vi "Write Bytes.vi"(8 "error in (no error)":errorcluster {"code" format="%.0x"}, 9 "Buffer":u32[](array[numeric])=[0], 10 "Count":i64 format="%.0g", 11 "instrument handle":refnum<k15>) -> (0 "error out":errorcluster {"code" format="%.0x"}, 2 "ReturnCount":i64, 3 "instrument handle out":refnum<k15>)   [LabVIEW 2020, in "Keysight DAQ970.lvlib"]
doc: "Write an array of bytes to the device."
uses:
  Keysight DAQ970.lvlib
  KtDAQ970.dll
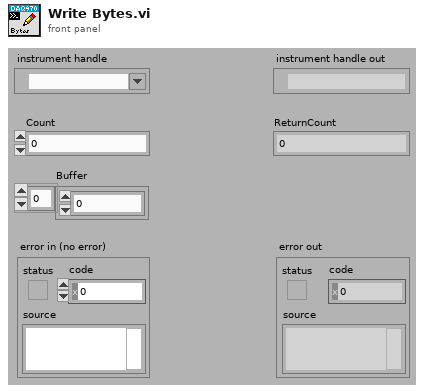
[diagram p1: front panel]
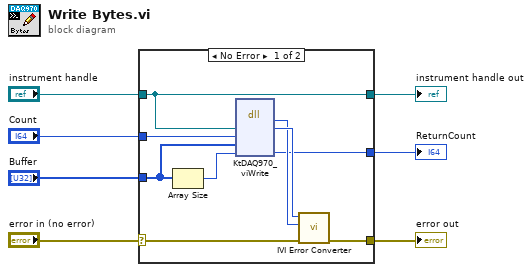
[diagram p0: block diagram]
diagram:
  n1 = case shown="No Error" "error in (no error)" {
    selector: "error in (no error)" -> [w14 w18]
    tunnel: [w13 w18] -> w7
    tunnel: "instrument handle" -> [w10 w17]
    tunnel: "Count" -> [w12 _]
    tunnel: "Buffer" -> [w9 _]
    tunnel: [w11 _] -> w3
    tunnel: [w10 w17] -> w2
    frame No Error {
      n2 = Array Size(array=w9) -> (size(s)=w8:i32)
      n3 = dll-call lib="KtDAQ970**.dll" fn="KtDAQ970_viWrite"("Vi"=w10, "Count"=w12, "Buffer"=w9, "ReturnCount"=w8) -> ("return type"=w15:i32, "Vi"=w16:u32, "ReturnCount"=w11:i64)  [unwired: 5 in, 2 out]
      n4 = call "IVI Error Converter.vi"("error in (no error)"=w14, "IVI error code (0)"=w15, "instrument handle"=w16) -> ("error out"=w13:errorcluster)  [unwired: 7 in, 1 out]
    }
    frame Error {
    }
  }
  "error out" <- w7
  "instrument handle out" <- w2
  "ReturnCount" <- w3
